vi "Disabled.vi"(7 "Robot Mode":T2, 10 "Match Info":T1={"Autonomous Elapsed Seconds"=0.0, "TeleOp Elapsed Seconds"=0.0, "Disabled Elapsed Seconds"=0.0, "Visited Autonomous"=FALSE, "Visited TeleOp"=FALSE, "Visited Disabled"=FALSE, "Autonomous Settings"={"Autonomous Style"=enum."Independent", "VI Refnum"=refnum}}, 11 "Call Context":T3) -> ()   [LabVIEW 2015]
doc: "This VI is called each time a disabled packet is received from the DS. It is often used to prepare for the next robot mode, to calibrate sensors, etc."
uses:
  Robot Global Data.vi
  Common Code/Catapult/Catapult Auto Commands.ctl
  Common Code/Intake Commands.ctl
  Common Code/Drivetrain Modes.ctl
  <vilib>/Rock Robotics/WPI/DriverStation/WPI_DriverStationRobotMode2.ctl
  <vilib>/Rock Robotics/WPI/DriverStation/WPI_DriverStationMatch Info.ctl
  <vilib>/Rock Robotics/WPI/DriverStation/WPI_DriverStationDerivedRobotMode.ctl
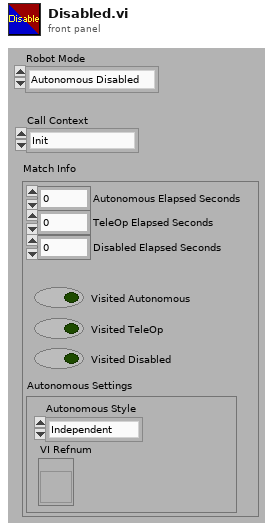
[diagram p1: front panel]
types:
  T1 = typedef "WPI_DriverStationMatch Info.ctl" = cluster{"Autonomous Elapsed Seconds":dbl, "TeleOp Elapsed Seconds":dbl, "Disabled Elapsed Seconds":dbl, "Visited Autonomous":bool, "Visited TeleOp":bool, "Visited Disabled":bool, "Autonomous Settings":cluster{"Autonomous Style":enum16{"Iterative", "Independent"}, "VI Refnum":refnum<vi>}}
  T2 = typedef "WPI_DriverStationRobotMode2.ctl" = enum16{"Autonomous Disabled", "Autonomous Enabled", "Teleop Disabled", "Teleop Enabled", "Disconnected", "Finish", "Test Disabled", "Test Enabled", "Emergency Stopped"}
  T3 = typedef "WPI_DriverStationDerivedRobotMode.ctl" = enum16{"Init", "Execute", "Stop"}
  T4 = typedef "Drivetrain Modes.ctl" = enum16{"Tank", "Climb", "Manual", "Goal Vision Targeting", "PID Distance Drive", "Hybrid", "Gyro Steer"}
  T5 = typedef "Intake Commands.ctl" = enum16{"Settle Ball", "Unload", "Load", "Pull up", "Drop low", "Idle", "Lift Half", "Go To Angle"}
  T6 = typedef "Catapult Auto Commands.ctl" = enum16{"Idle", "Warmup", "Shoot"}
  T7 = typedef "Drivetrain Commands.ctl" = cluster{"Y Power":dbl, "Turn Power":dbl, "Modes":T4, "Heading Target":dbl, "X Max Speed":dbl, "Y Max Speed":dbl, "X Min Speed":dbl, "Y Min Speed":dbl, "Y Target":dbl, "Max Accel":dbl, "Max Velocity":dbl, "Y Power 2":dbl, "Pivot Speed":dbl}
  T8 = typedef "WPI_JoystickDevRef.ctl" = cluster{"Device":T9}
  T9 = typedef "WPI_JoystickDeviceEnum.ctl" = enum16{"USB 0", "USB 1", "USB 2", "USB 3", "USB 4", "USB 5"}
  T10 = typedef "Intake Mode.ctl" = enum16{"Safe", "Auto", "Manual"}
  T11 = typedef "Intake Commands Cluster.ctl" = cluster{"Intake Commands":T5, "Intake Mode":T10, "Override IR":bool, "Angle Target":dbl}
  T12 = typedef "Climb Command Cluster.ctl" = cluster{"Climb Mode":T13, "Hold?":bool, "Manual State":T14}
  T13 = typedef "Climb Mode.ctl" = enum16{"Auto", "Semi-Auto", "Manual"}
  T14 = typedef "Climb Manual State.ctl" = cluster{"Release":bool, " PTO Engage":bool, "Extend":bool}
  T15 = typedef "D-Pad.ctl" = cluster{"Top":bool, "Bottom":bool, "None":bool, "Right":bool, "Left":bool}
  T16 = typedef "Button Cluster.ctl" = cluster{"Buttons[0]":bool, "Buttons[1]":bool, "Buttons[2]":bool, "Buttons[3]":bool, "Buttons[4]":bool, "Buttons[5]":bool, "Buttons[6]":bool, "Buttons[7]":bool, "Buttons[8]":bool, "Buttons[9]":bool}
  T17 = typedef "Shooter Command Cluster.ctl" = cluster{"Command":T6, "Mode":T18, "Shot Type":T19, "Override Trigger Sensor":bool, "Override Angle?":bool, "Hide From Death":bool}
  T18 = typedef "Shoot Modes Enum.ctl" = enum16{"Manual", "Auto"}
  T19 = typedef "Shot Type.ctl" = enum16{"Batter Shot", "Corner Shot", "Cleat Shot", "Vision Shot", "Deep Middle Shot"}
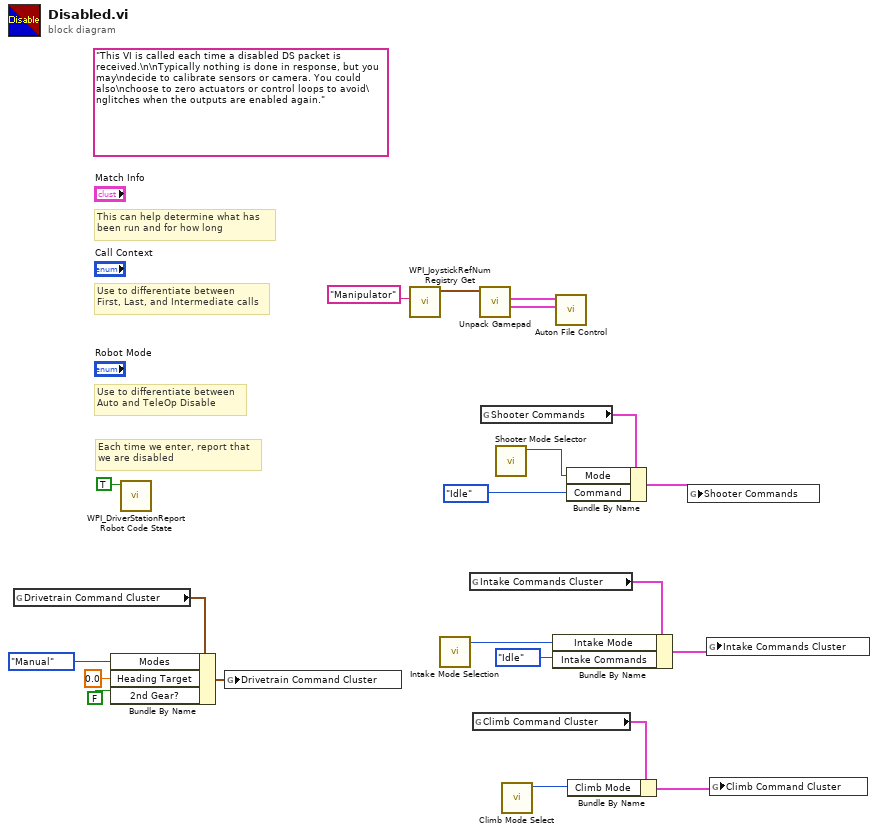
[diagram p0: block diagram]
diagram:
  (unwired) "This VI is called each time a disabled DS packet is received.\n\nTypically nothing is done in response, but you may\ndecide to calibrate sensors or camera. You could also\nchoose to zero actuators or control loops to avoid\nglitches when the outputs are enabled again."
  # "Each time we enter, report that\nwe are disabled"
  # "Use to differentiate between\nFirst, Last, and Intermediate calls"
  # "This can help determine what has\nbeen run and for how long"
  # "Use to differentiate between\nAuto and TeleOp Disable"
  n1 = global read "Robot Global Data.vi" "Drivetrain Command Cluster"() -> (w5:T7)
  n2 = Bundle By Name(cluster=w5, "Modes"=Drivetrain_Modes."Manual", "Heading Target"=0.0, "2nd Gear?"=FALSE) -> (w4:T7)
  n3 = call <vilib>:"WPI_DriverStationReport Robot Code State.vi"("Disabled"=TRUE ("Autonomous")) -> ()  [unwired: 10 in, 1 out]
  n4 = global write "Robot Global Data.vi" "Drivetrain Command Cluster"(w4) -> ()
  n5 = call <vilib>:"WPI_JoystickRefNum Registry Get.vi"("refnum name"="Manipulator") -> ("JoystickDevRef"=w19:T8)  [unwired: 1 in, 9 out]
  n6 = call "Intake Mode Selection.vi"() -> ("Mode"=w9:T10)  [unwired: 11 in]
  n7 = global read "Robot Global Data.vi" "Intake Commands Cluster"() -> (w11:T11)
  n8 = global read "Robot Global Data.vi" "Climb Command Cluster"() -> (w8:T12)
  n9 = call "Unpack Gamepad.vi"("JoystickDevRef"=w19) -> ("D-Pad"=w17:T15, "Button Cluster"=w18:T16)  [unwired: 8 in, 1 out]
  n10 = global read "Robot Global Data.vi" "Shooter Commands"() -> (w16:T17)
  n11 = call "Shooter Mode Selector.vi"() -> ("Mode"=w15:T18)  [unwired: 11 in]
  n12 = call "Climb Mode Select.vi"() -> ("Mode"=w6:T13)  [unwired: 11 in]
  n13 = Bundle By Name(cluster=w11, "Intake Mode"=w9, "Intake Commands"=Intake_Commands."Idle") -> (w12:T11)
  n14 = call "Auton File Control.vi"("Manip D-Pad"=w17, "Manip Button"=w18) -> ()  [unwired: 10 in]
  n15 = Bundle By Name(cluster=w16, "Mode"=w15, "Command"=Catapult_Auto_Commands."Idle") -> (w13:T17)
  n16 = Bundle By Name(cluster=w8, "Climb Mode"=w6) -> (w7:T12)
  n17 = global write "Robot Global Data.vi" "Shooter Commands"(w13) -> ()
  n18 = global write "Robot Global Data.vi" "Intake Commands Cluster"(w12) -> ()
  n19 = global write "Robot Global Data.vi" "Climb Command Cluster"(w7) -> ()
